vi "compare readings R140.vi"() -> ()   [LabVIEW 2020]
uses:
  file handler/VFH-VNA_File_Handler.lvlib
panel:
  in  "Tab Control":enum32{"Page 1", "Page 3", "Page 2"}(tab)
  in  "Max range":dbl
  in  "min range":dbl
  out "Ref R":cluster{"Frequency":dbl[], "S21_Imag":dbl[]}[](graph)
  out "Ref I":cluster{"Frequency":dbl[], "S21_Imag":dbl[]}[](graph)
  out "p'":cluster{"Frequency":dbl[], "S21_Imag":dbl[]}[](graph)
  out "p''":cluster{"Frequency":dbl[], "S21_Imag":dbl[]}[](graph)
  in  "Stop":bool
  in  "Max range 2":dbl
  in  "min range 2":dbl
  out "Tan":cluster{"Frequency":dbl[], "S21_Imag":dbl[]}[](graph)
  out "Q [S/m]":cluster{"Frequency":dbl[], "S21_Imag":dbl[]}[](graph)
  in  "Stop 2":bool
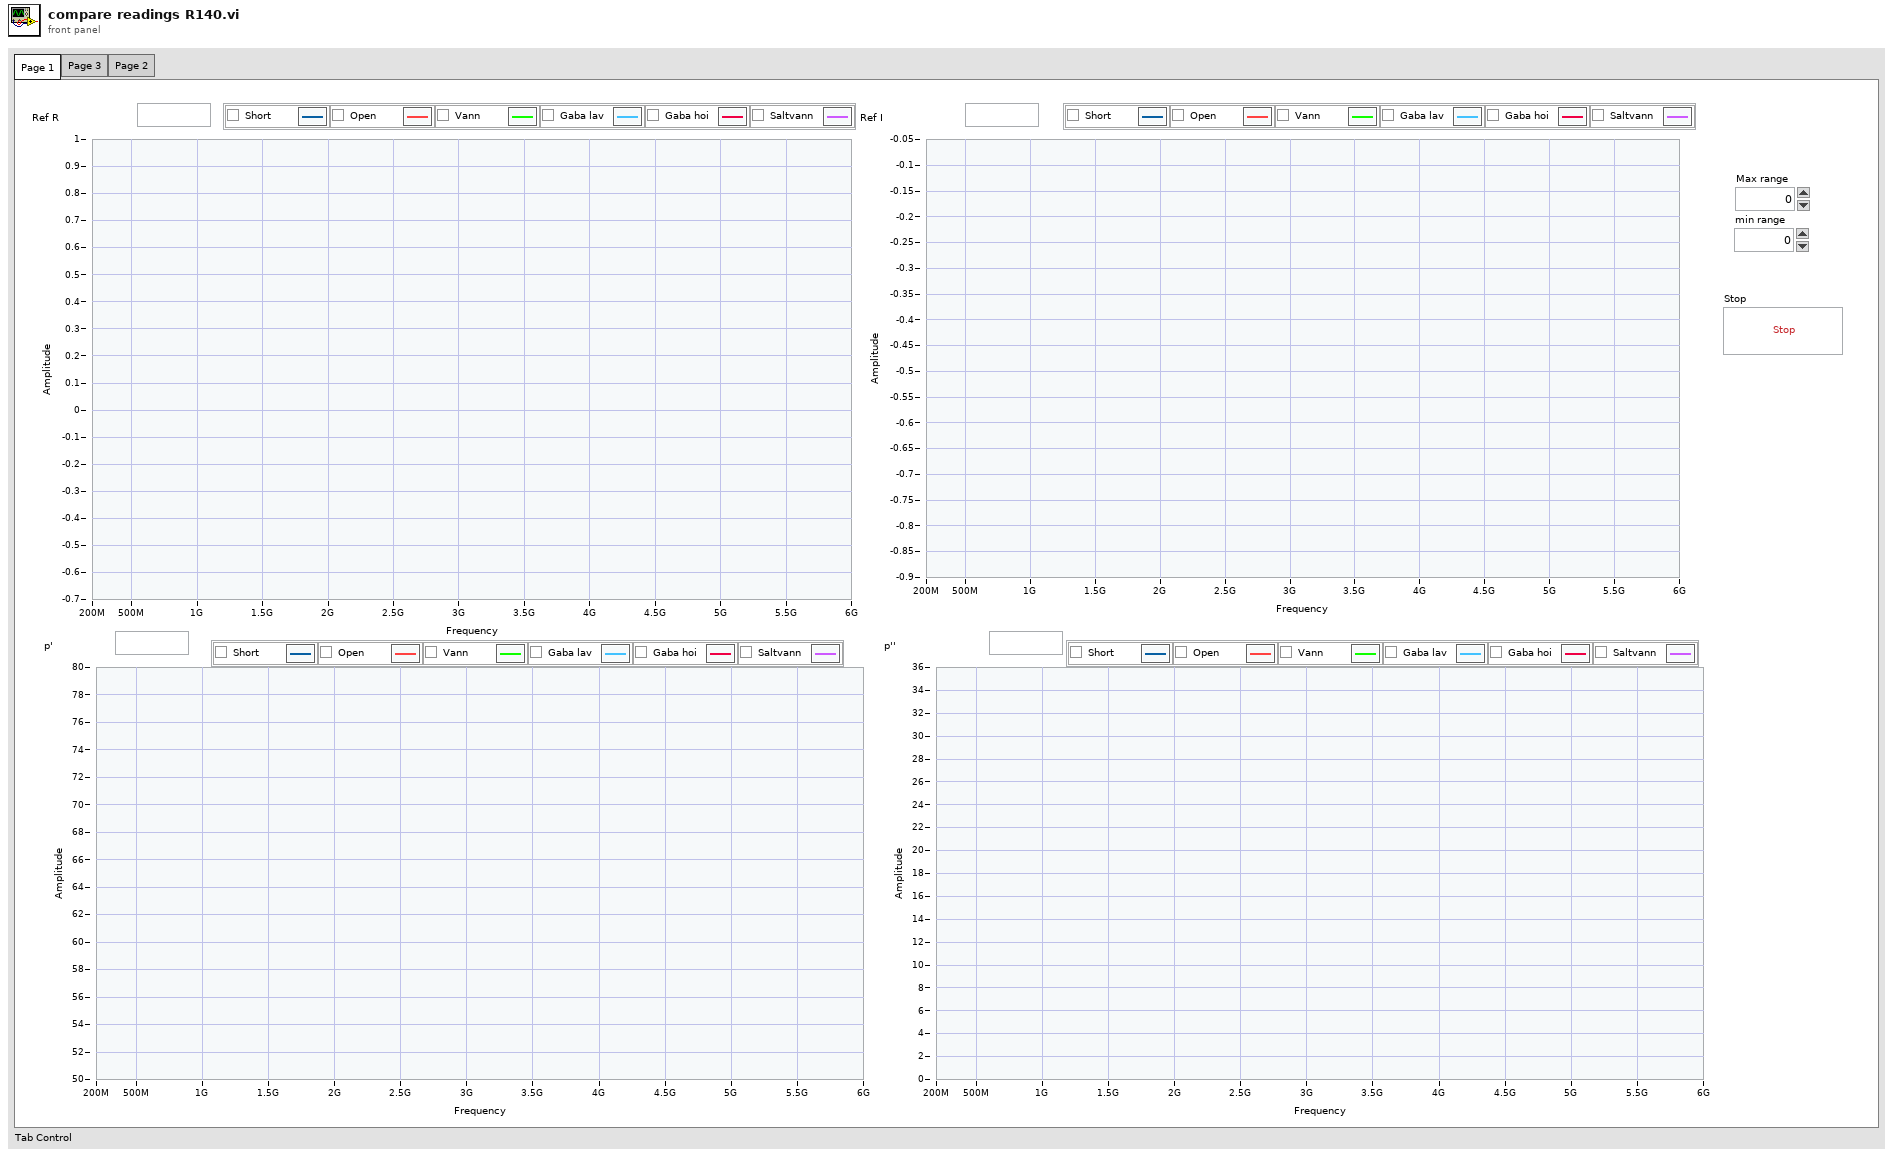
[diagram p1: front panel]
types:
  T1 = typedef "VFH-VNA_File_Handler.lvlib/VFH-file_cluster-Expensive.ctl" = cluster{"Frequency":dbl[], "Permativity'":dbl[], "Permativity''":dbl[], "Q [S/m]":dbl[], "Tan":dbl[], "Reflection R":dbl[], "Reflection I":dbl[]}
  T2 = cluster{"Frequency":dbl[], "Permativity''":dbl[]}
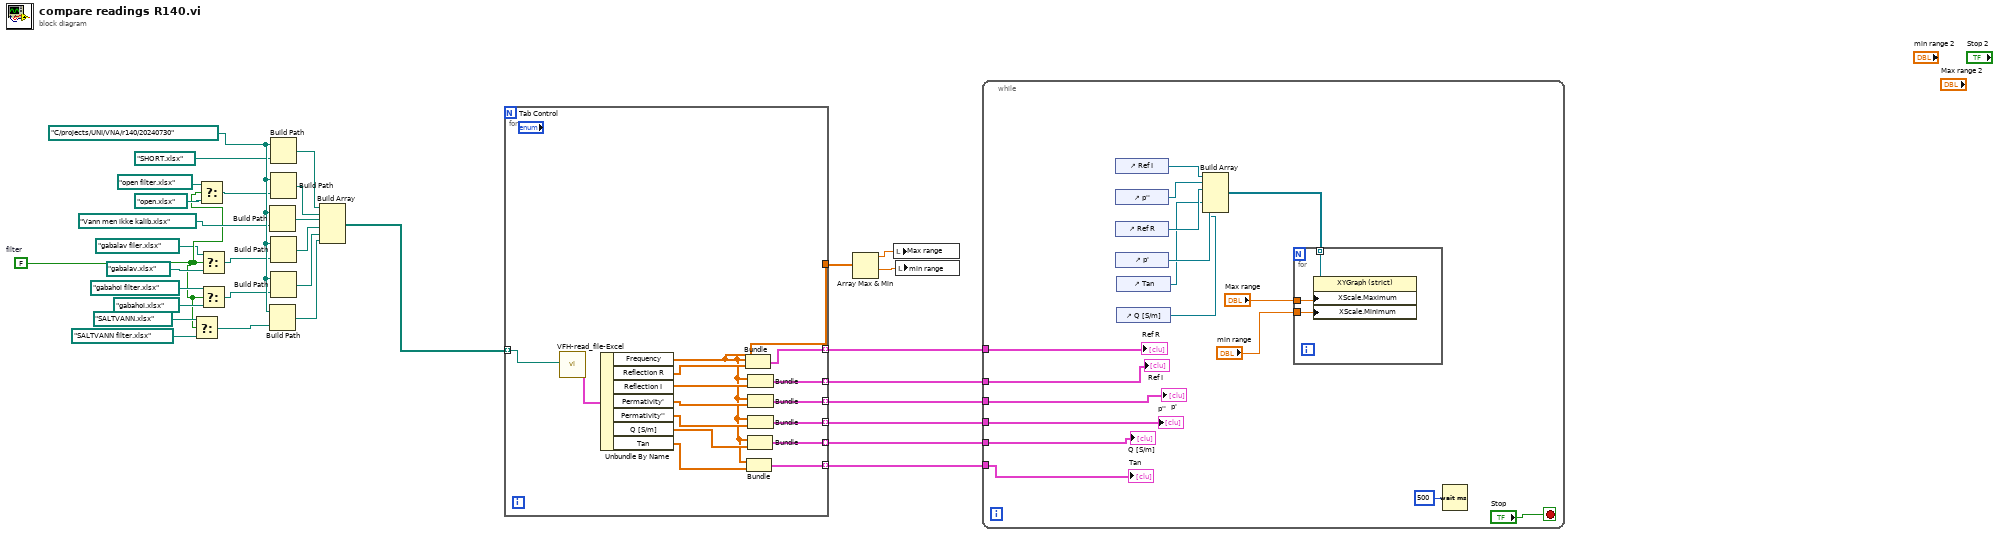
[diagram p0: block diagram]
diagram:
  w3 = FALSE  # filter
  w17 = path "C:/projects/UNI/VNA/r140/20240730" ("Folder Path")
  n1 = Select(t=path "SALTVANN.xlsx" ("name or relative path"), s=w3, f=path "SALTVANN filter.xlsx" ("name or relative path")) -> (s? t:f=w7:path)
  n2 = Select(t=path "open filter.xlsx" ("name or relative path"), s=w3, f=path "open.xlsx" ("name or relative path")) -> (s? t:f=w5:path)
  n3 = Select(t=path "gabalav filer.xlsx" ("name or relative path"), s=w3, f=path "gabalav.xlsx" ("name or relative path")) -> (s? t:f=w2:path)
  n4 = Select(t=path "gabahoi filter.xlsx" ("name or relative path"), s=w3, f=path "gabahoi.xlsx" ("name or relative path")) -> (s? t:f=w10:path)
  n5 = Build Path(base path=w17, name or relative path=path "Vann men ikke kalib.xlsx") -> (appended path=w21:path)
  n6 = Build Path(base path=w17, name or relative path=w7) -> (appended path=w18:path)
  n7 = Build Path(base path=w17, name or relative path=path "SHORT.xlsx") -> (appended path=w23:path)
  n8 = Build Path(base path=w17, name or relative path=w5) -> (appended path=w22:path)
  n9 = Build Path(base path=w17, name or relative path=w2) -> (appended path=w20:path)
  n10 = Build Path(base path=w17, name or relative path=w10) -> (appended path=w19:path)
  n11 = Build Array(w23, w22, w21, w20, w19, w18) -> (w15:path[])
  n12 = for {
    tunnel: w15 -> [w47] mode=indexing
    tunnel: [w41] -> w32 mode=indexing
    tunnel: [w40] -> w31 mode=indexing
    tunnel: [w39] -> w30 mode=indexing
    tunnel: [w38] -> w29 mode=indexing
    tunnel: [w35] -> w28
    tunnel: [w34] -> w25 mode=indexing
    tunnel: [w33] -> w24 mode=indexing
    n13 = call "VFH-read_file-Excel.vi"("file path (dialog if empty)"=w47) -> ("output cluster"=w46:T1)  [unwired: 9 in, 1 out]
    n14 = Unbundle By Name(w46) -> ("Frequency"=w35:dbl[], "Reflection R"=w45:dbl[], "Reflection I"=w44:dbl[], "Permativity'"=w43:dbl[], "Permativity''"=w42:dbl[], "Q [S/m]"=w36:dbl[], "Tan"=w37:dbl[])
    n15 = Bundle("Frequency"=w35, "Reflection R"=w45) -> (w41:cluster{"Frequency":dbl[], "Reflection R":dbl[]})  [unwired: 1 in]
    n16 = Bundle("Frequency"=w35, "Tan"=w37) -> (w33:cluster{"Frequency":dbl[], "Tan":dbl[]})  [unwired: 1 in]
    n17 = Bundle("Frequency"=w35, "Q [S/m]"=w36) -> (w34:cluster{"Frequency":dbl[], "Q [S/m]":dbl[]})  [unwired: 1 in]
    n18 = Bundle("Frequency"=w35, "Reflection I"=w44) -> (w40:cluster{"Frequency":dbl[], "Reflection I":dbl[]})  [unwired: 1 in]
    n19 = Bundle("Frequency"=w35, "Permativity'"=w43) -> (w39:cluster{"Frequency":dbl[], "Permativity'":dbl[]})  [unwired: 1 in]
    n20 = Bundle("Frequency"=w35, "Permativity''"=w42) -> (w38:T2)  [unwired: 1 in]
  }
  n21 = Array Max & Min(array=w28) -> (max value=w27:dbl, min value=w26:dbl)  [unwired: 2 out]
  n22 = local write "Max range"(w27) -> ()
  n23 = local write "min range"(w26) -> ()
  n24 = while {
    tunnel: w32 -> [w62]
    tunnel: w31 -> [w61]
    tunnel: w30 -> [w60]
    tunnel: w29 -> [w59]
    tunnel: w25 -> [w51]
    tunnel: w24 -> [w50]
    stop <- "Stop" stop-if-true
    n25 = control-ref of="Ref I"() -> (w58:refnum<vi>)
    n26 = control-ref of="p''"() -> (w57:refnum<vi>)
    n27 = control-ref of="Ref R"() -> (w56:refnum<vi>)
    n28 = control-ref of="p'"() -> (w55:refnum<vi>)
    n29 = control-ref of="Tan"() -> (w49:refnum<vi>)
    n30 = control-ref of="Q [S/m]"() -> (w48:refnum<vi>)
    n31 = Build Array(w58, w57, w56, w55, w49, w48) -> (w54:refnum<vi>[])
    n32 = for {
      tunnel: w54 -> [w67] mode=indexing
      tunnel: "Max range" -> [w66]
      tunnel: "min range" -> [w65]
      n33 = property class="XYGraph (strict)"(reference=w67, "XScale.Maximum"=w66, "XScale.Minimum"=w65) -> ()  [unwired: 1 in, 2 out]
    }
    n34 = Wait (ms)(milliseconds to wait=u32 500) -> ()  [unwired: 1 out]
    "p'" <- w60
    "Ref R" <- w62
    "p''" <- w59
    "Ref I" <- w61
    "Q [S/m]" <- w51
    "Tan" <- w50
  }
